vi "MEMR-Restore Defaults.vi"() -> (8 "Params":T1={"Probe"={"Ear"=enum."Right", "Stimulus"=enum."Click", "Duration (us)"=100.0, "Level"=90.0}, "Elicitor"={"Duration (ms)"=100.0, "Ramp (ms)"=2.5, "Transducer"=enum."Insert"}, "Sequence"={"Start"=40.0, "Stop"=92.0, "Step"=4.0}, "Analysis"={"T(ms) re peak"=2.0, "Fmin (Hz)"=800.0, "Fmax (Hz)"=3200.0, "Window"=enum."Hamming", "Gain (dB)"=40.0, "Resol (Hz)"=0.0}, "Repeats"=2, "Timing"={"Click1-Noise (ms)"=30.0, "Noise-Click2 (ms)"=5.0, "ISI (ms)"=1135.0}, "Save raw"=FALSE, "Fs (Hz)"=50000.0})   [LabVIEW 2020]
uses:
  Typedefs/MEMR-Params.ctl
  Typedefs/MEMR-Probe.ctl
  Typedefs/MEMR-Elicitor.ctl
  Human Studies/SFM Frontend/LV Source/Typedefs/HSTS-Transducer.ctl
  Typedefs/MEMR-Sequence.ctl
  Typedefs/MEMR-Analysis.ctl
  Typedefs/MEMR-Timing.ctl
panel:
  out "error out":errorcluster
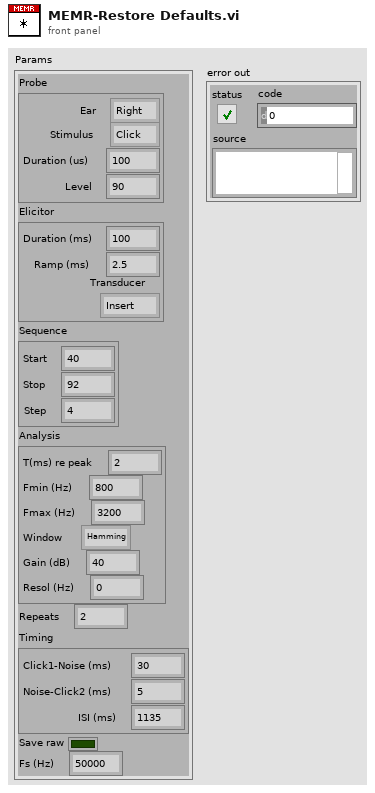
[diagram p1: front panel]
types:
  T1 = typedef "MEMR-Params.ctl" = cluster{"Probe":T2, "Elicitor":T3, "Sequence":T5, "Analysis":T6, "Repeats":i32, "Timing":T7, "Save raw":bool, "Fs (Hz)":dbl}
  T2 = typedef "MEMR-Probe.ctl" = cluster{"Ear":enum16{"Right", "Left"}, "Stimulus":enum16{"Click", "Chirp"}, "Duration (us)":dbl, "Level":dbl}
  T3 = typedef "MEMR-Elicitor.ctl" = cluster{"Duration (ms)":dbl, "Ramp (ms)":dbl, "Transducer":T4}
  T4 = typedef "HSTS-Transducer.ctl" = enum16{"Insert", "TDH-39", "HD300", "ER-10X"}
  T5 = typedef "MEMR-Sequence.ctl" = cluster{"Start":dbl, "Stop":dbl, "Step":dbl}
  T6 = typedef "MEMR-Analysis.ctl" = cluster{"T(ms) re peak":dbl, "Fmin (Hz)":dbl, "Fmax (Hz)":dbl, "Window":enum16{"None", "Hanning", "Hamming"}, "Gain (dB)":dbl, "Resol (Hz)":dbl}
  T7 = typedef "MEMR-Timing.ctl" = cluster{"Click1-Noise (ms)":dbl, "Noise-Click2 (ms)":dbl, "ISI (ms)":dbl}
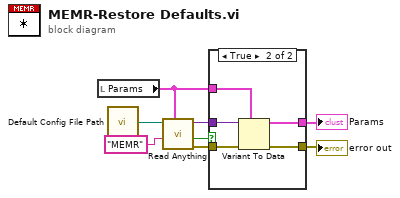
[diagram p0: block diagram]
diagram:
  n1 = local read "Params"() -> (w3:T1)
  n2 = call "Default Config File Path.vi"() -> ("Default config file name"=w8:path)
  n3 = call "Read Anything.vi"("Type of Anything"=w3, "Section Name (Name of \"Type of Anything\")"="MEMR" ("Section Name (Name of \"Type of Anything\")"), "Path (dialog)"=w8) -> ("Error Out"=w5:errorcluster, "Found?"=w4:bool, "Anything"=w6:variant)  [unwired: 6 in]
  n4 = case shown="True" w4 {
    tunnel: w6 -> [_ w14]
    tunnel: w5 -> [w9 w15]
    tunnel: w3 -> [w10 w13]
    tunnel: [w10 w12] -> w2
    tunnel: [w9 w11] -> w1
    frame False {
    }
    frame True {
      n5 = Variant To Data(error in=w15, type=w13, Variant=w14) -> (data=w12:T1, error out=w11:errorcluster)
    }
  }
  "Params" <- w2
  "error out" <- w1
